vi "Keys.vi"(8 "error in (no error)":errorcluster, 11 "VariantAttribute in":refnum<class "MapImp.lvclass">) -> (0 "error out":errorcluster, 2 "Keys":string[](array[string]), 3 "VariantAttribute out":refnum<class "MapImp.lvclass">)   [LabVIEW 2013, in "LapDog.Collections.v_.Maps.lvlib" / "MapImp.lvclass"]
doc: "Returns a copy of all keys in the map."
uses:
  MapImp.lvclass
  MapImp.lvclass/MapImp.ctl
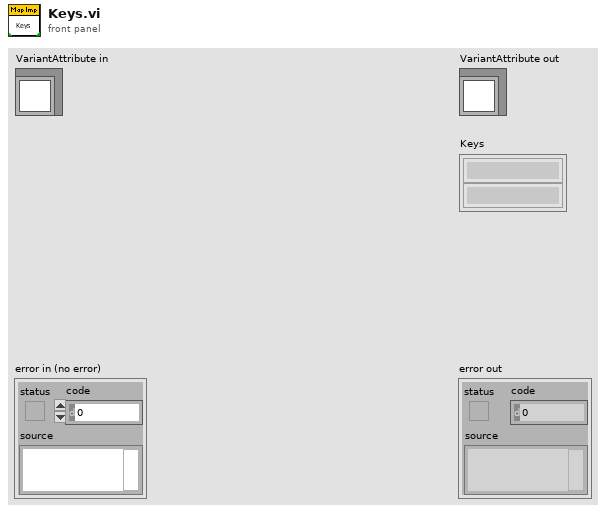
[diagram p1: front panel]
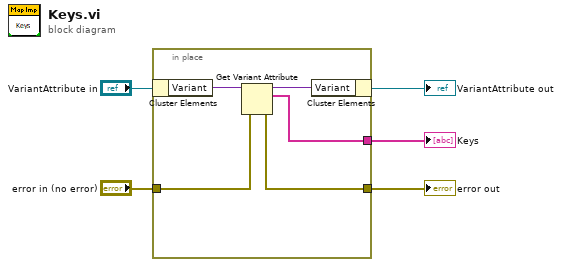
[diagram p0: block diagram]
diagram:
  n1 = in-place {
    in-place-border: "error in (no error)" -> [w9]
    in-place-border: [w8] -> w3
    in-place-border: [w6] -> w2
    n2 = in-place-cluster #1("VariantAttribute in") -> ("Variant"=w10:variant)
    n3 = Get Variant Attribute(Variant=w10, error in=w9) -> (duplicate Variant=w7:variant, names=w6:string[], error out=w8:errorcluster)  [unwired: 2 in, 1 out]
    n4 = in-place-cluster #1("Variant"=w7) -> (→"VariantAttribute out":refnum<class "MapImp.lvclass">)
  }
  "error out" <- w3
  "Keys" <- w2
